vi "Test Assert Equal (Float Units).vi"(8 "error in (no error)":errorcluster) -> (0 "error out":errorcluster)   [LabVIEW 2009]
uses:
  classes/Test/Test.lvclass
  classes/Assert/Assert.lvclass
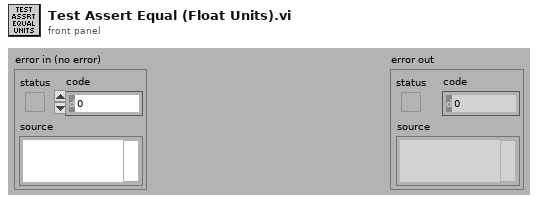
[diagram p1: front panel]
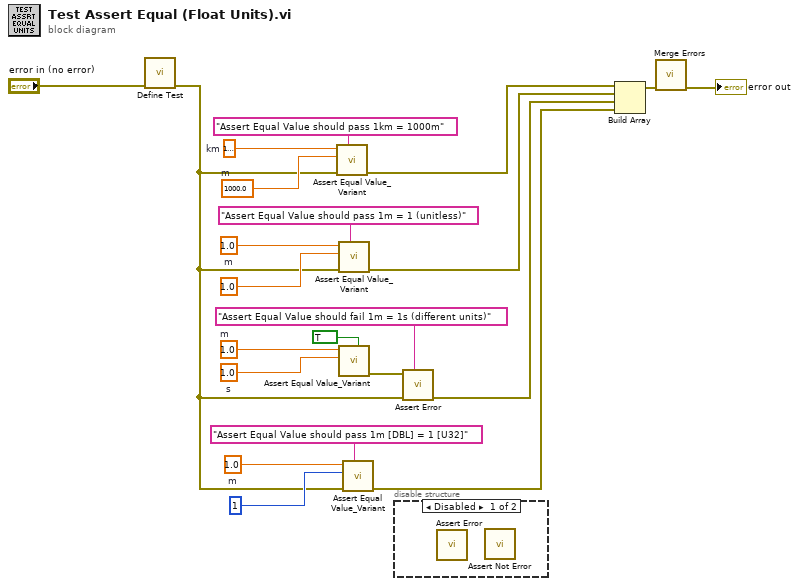
[diagram p0: block diagram]
diagram:
  w5 = dbl[unit] 1.0  # m
  w10 = dbl[unit] 1.0  # s
  w11 = dbl[unit] 1.0  # m
  w13 = dbl[unit] 1.0  # m
  w18 = dbl[unit] 1000.0  # m
  w19 = dbl[unit] 1000.0  # km
  n1 = call "Define Test.vi"("error in (no error)"="error in (no error)") -> ("error out"=w2:errorcluster)  [unwired: 10 in]
  n2 = call "Assert Equal Value_Variant.vi"("Label"="Assert Equal Value should pass 1km = 1000m", "error in (no error)"=w2, "Y"=w18, "X"=w19) -> ("error out"=w17:errorcluster)  [unwired: 7 in]
  n3 = call "Assert Equal Value_Variant.vi"("Label"="Assert Equal Value should pass 1m = 1 (unitless)", "error in (no error)"=w2, "Y"=1.0, "X"=w13) -> ("error out"=w12:errorcluster)  [unwired: 7 in]
  n4 = call "Assert Equal Value_Variant.vi"("Assert Only? (F)"=TRUE, "Y"=w10, "X"=w11) -> ("error out"=w7:errorcluster)  [unwired: 8 in]
  n5 = call "Assert Equal Value_Variant.vi"("Label"="Assert Equal Value should pass 1m [DBL] = 1 [U32]", "error in (no error)"=w2, "Y"=u32 1, "X"=w5) -> ("error out"=w1:errorcluster)  [unwired: 7 in]
  n6 = disable-structure shown="Disabled" {
    frame #0 {
      n7 = call "Assert Error.vi"() -> ()  [unwired: 11 in, 1 out]
      n8 = call "Assert Not Error.vi"() -> ()  [unwired: 11 in, 1 out]
    }
    frame #1 {
    }
  }
  n9 = call "Assert Error.vi"("Label"="Assert Equal Value should fail 1m = 1s (different units)", "error in (no error)"=w2, "Error?"=w7) -> ("error out"=w6:errorcluster)  [unwired: 8 in]
  n10 = Build Array(w17, w12, w6, w1) -> (w20:errorcluster[])
  n11 = call <vilib>:"Merge Errors.vi"("error array in"=w20) -> ("error out"=→"error out":errorcluster)  [unwired: 6 in]
